vi "Write.vi"(8 "error in (no error)":errorcluster, 9 "Start address":string, 10 "Read Type":variant, 11 "MelsecTCP in":refnum<class "InovanceSerial.lvclass">) -> (0 "error out":errorcluster, 3 "MelsecTCP out":refnum<class "InovanceSerial.lvclass">)   [LabVIEW 2020, in "HslCommunication.lvlib" / "InovanceSerial.lvclass"]
uses:
  InovanceSerial.lvclass
  D:/Git/Labview-Libraries/Libraries/HslCommunication/Abstract PLC Controler/Abstract PLC Controler.lvclass
  EventLogger.lvlibp/1abvi3w/vi.lib/gpm_packages/@cs/event-logger/Source/Composed Log/Types/Log Level.ctl
  Abstract PLC Controler/Abstract PLC Controler.lvclass/Abstract PLC Controler.ctl
  D:/Git/Labview-Libraries/Libraries/HslCommunication/_Dependenciecs/HslCommunication.dll
  _Dependenciecs/HslCommunication.dll
  Read reference.vi
  Abstract PLC Controler/Abstract PLC Controler.lvclass
  InovanceSerial.lvclass/InovanceSerial.ctl
  <vilib>/Utility/Data Type/NI_Data Type.lvlib
  EventLogger.lvlibp/Logger.lvclass
  EventLogger.lvlibp/1abvi3w/vi.lib/gpm_packages/@cs/event-logger/Source/Composed Log/Composed Log.lvlib
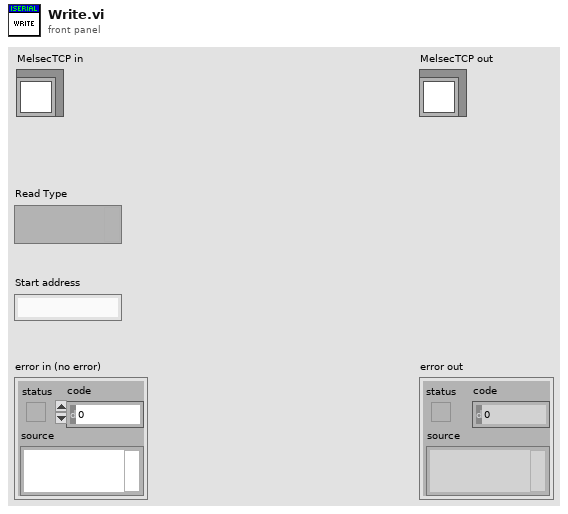
[diagram p1: front panel]
types:
  T1 = typedef "EventLogger.lvlibp/Composed Log.lvlib/Log Level.ctl" = enum16{"Debug", "Info", "Warning", "Error", "Critical"}
  T2 = typedef "NI_Data Type.lvlib/Data Type.ctl" = enum8{"Invalid Type", "Void", "I8", "I16", "I32", "I64", "U8", "U16", "U32", "U64", "Single Float", "Double Float", "Extended Float", "Single Complex", "Double Complex", "Extended Complex", "Enum U8", "Enum U16", "Enum U32", "Enum U64", "Single Float With Unit", "Double Float With Unit", "Extended Float With Unit", "Single Complex with Unit", "Double Complex with Unit", "Extended Complex with Unit", "Boolean", "String", "Path", "Picture", "Tag", "Array", "Cluster", "Variant", "LV Variant", "Waveform", "Timestamp", "Digital Waveform", "Digital Data", "ExpressData", "Refnum", "External Data", "VI", "Poly VI", "LabVIEW Class Instance", "Fixed Point", "Set Collection", "Map Collection"}
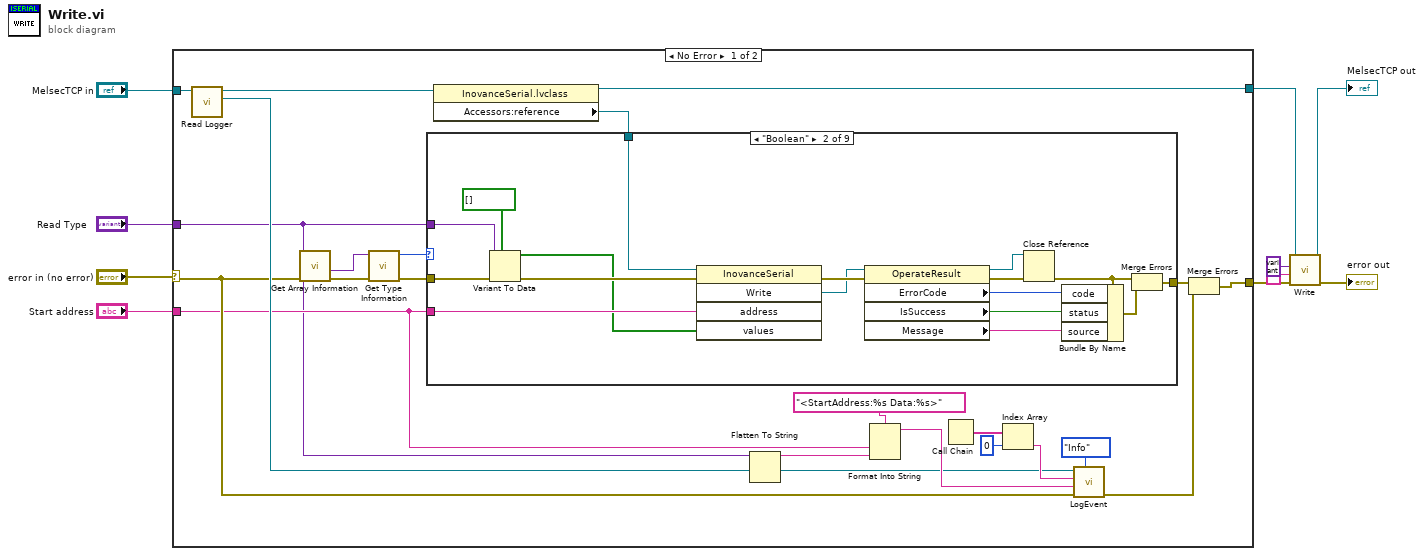
[diagram p0: block diagram]
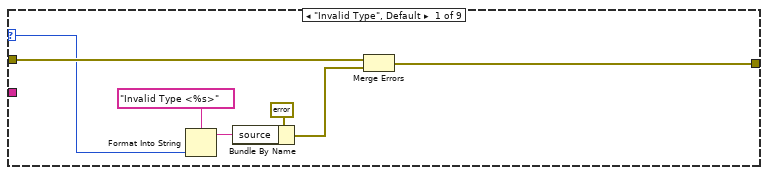
[diagram p2: hidden frame]
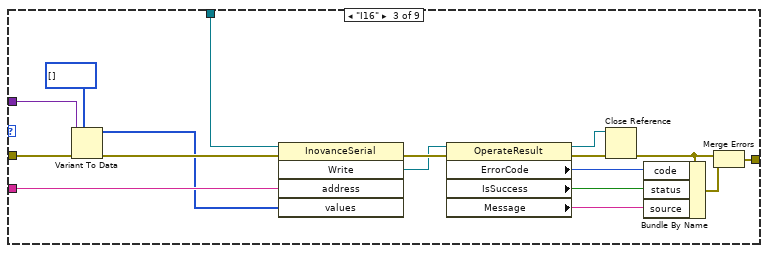
[diagram p3: hidden frame]
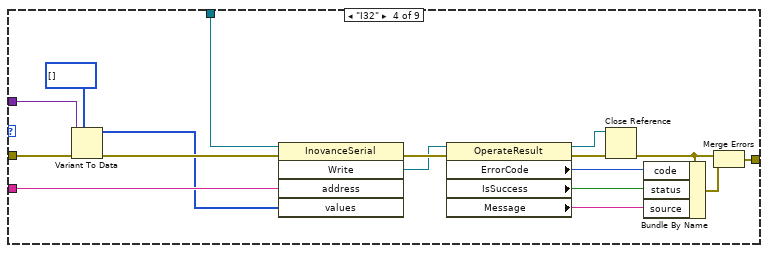
[diagram p4: hidden frame]
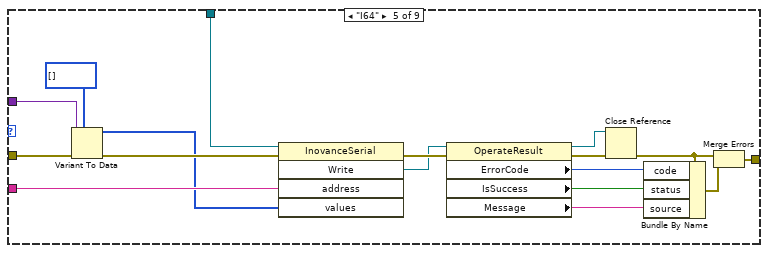
[diagram p5: hidden frame]
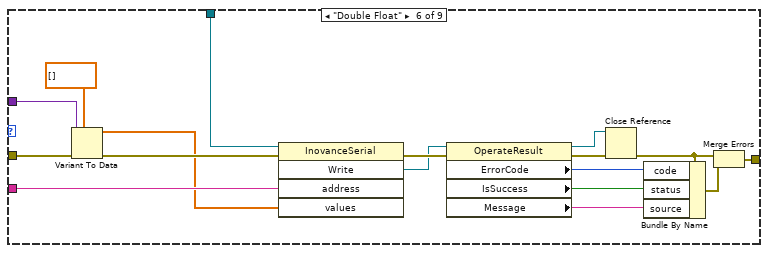
[diagram p6: hidden frame]
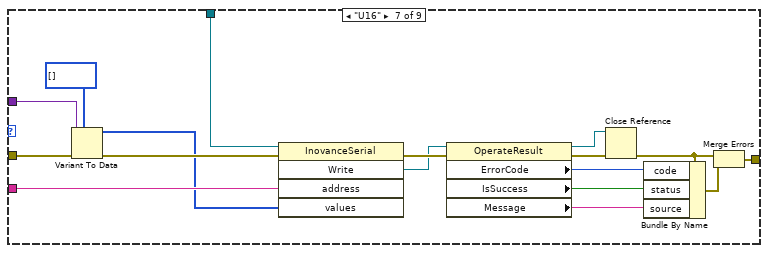
[diagram p7: hidden frame]
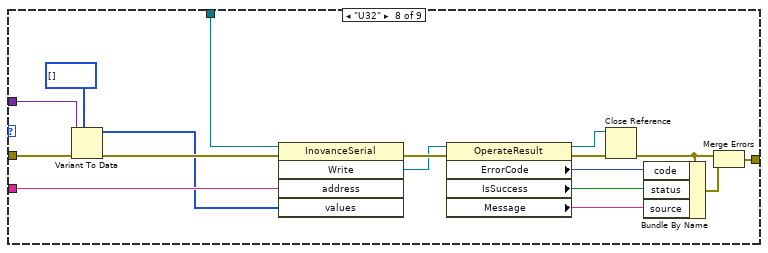
[diagram p8: hidden frame]
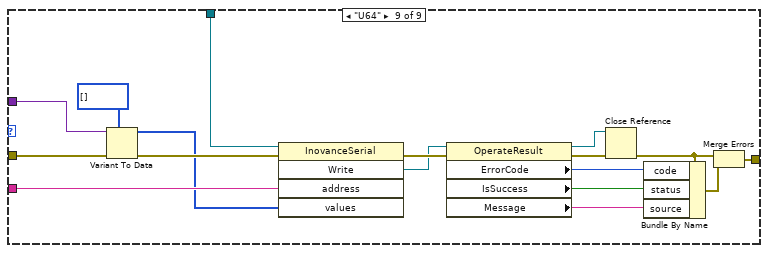
[diagram p9: hidden frame]
diagram:
  n1 = case shown="No Error" "error in (no error)" {
    selector: "error in (no error)" -> [w16 w177]
    tunnel: "MelsecTCP in" -> [w32 w176]
    tunnel: [w29 w176] -> w4
    tunnel: "Start address" -> [w15 _]
    tunnel: [w12 w177] -> w7
    tunnel: "Read Type" -> [w14 _]
    frame No Error {
      n2 = call "Read Logger.vi"("Abstract PLC Controler in"=w32) -> ("EventLogger.lvlibp:Logger.lvclass"=w17:refnum<class "Logger.lvclass">, "Abstract PLC Controler out"=w18:refnum<class "InovanceSerial.lvclass">)  [unwired: 9 in]
      n3 = call <vilib>:"Get Array Information.vi"("error in (no error)"=w16, "variant"=w14) -> ("error out"=w27:errorcluster, "array element data type"=w28:variant)  [unwired: 6 in, 2 out]
      n4 = call <vilib>:"Get Type Information.vi"("error in (no error)"=w27, "variant"=w28) -> ("error out"=w26:errorcluster, "type"=w25:T2)  [unwired: 5 in, 3 out]
      n5 = property class="InovanceSerial.lvclass"(reference=w18) -> (reference out=w29:refnum<class "InovanceSerial.lvclass">, "Accessors:reference"=w31:refnum<k24>)  [unwired: 1 in, 1 out]
      n6 = case shown="\"Boolean\"" w25 {
        selector: w25 -> [w37 _ _ _ _ _ _ _ _]
        tunnel: w31 -> [_ w56 w73 w90 w107 w124 w141 w158 w175]
        tunnel: w15 -> [_ w55 w72 w89 w106 w123 w140 w157 w174]
        tunnel: [w38 w54 w71 w88 w105 w122 w139 w156 w173] -> w30
        tunnel: w14 -> [_ w48 w65 w82 w99 w116 w133 w150 w167]
        tunnel: w26 -> [w39 w47 w64 w81 w98 w115 w132 w149 w166]
        frame "Invalid Type", Default {
          n7 = Format Into String(format string="Invalid Type <%s>", w37) -> (resulting string=w34:string)  [unwired: 2 in, 1 out]
          n8 = Bundle By Name(cluster=errorcluster {"status"=TRUE, "code"=-1, "source"=""} ("error IO"), "source"=w34) -> (w33:errorcluster)
          n9 = Merge Errors(w39, w33) -> (w38:errorcluster)
        }
        frame "Boolean" {
          n10 = Variant To Data(error in=w47, type=bool[] [], Variant=w48) -> (data=w40:bool[], error out=w42:errorcluster)
          n11 = invoke class="InovanceSerial" method="Write"(reference=w56, error in=w42, "address"=w55, "values"=w40) -> (error out=w46:errorcluster, "Write"=w44:refnum<k24>)  [unwired: 1 in, 3 out]
          n12 = property class="OperateResult"(reference=w44, error in=w46) -> (reference out=w43:refnum<k24>, error out=w45:errorcluster, "ErrorCode"=w53:i32, "IsSuccess"=w52:bool, "Message"=w51:string)
          n13 = Close Reference(reference=w43, error in (no error)=w45) -> (error out=w50:errorcluster)
          n14 = Bundle By Name(cluster=w50, "code"=w53, "status"=w52, "source"=w51) -> (w49:errorcluster)
          n15 = Merge Errors(w50, w49) -> (w54:errorcluster)
        }
        frame "I16" {
          n16 = Variant To Data(error in=w64, type=i16[] [], Variant=w65) -> (data=w57:i16[], error out=w59:errorcluster)
          n17 = invoke class="InovanceSerial" method="Write"(reference=w73, error in=w59, "address"=w72, "values"=w57) -> (error out=w63:errorcluster, "Write"=w61:refnum<k24>)  [unwired: 1 in, 3 out]
          n18 = property class="OperateResult"(reference=w61, error in=w63) -> (reference out=w60:refnum<k24>, error out=w62:errorcluster, "ErrorCode"=w70:i32, "IsSuccess"=w69:bool, "Message"=w68:string)
          n19 = Close Reference(reference=w60, error in (no error)=w62) -> (error out=w67:errorcluster)
          n20 = Bundle By Name(cluster=w67, "code"=w70, "status"=w69, "source"=w68) -> (w66:errorcluster)
          n21 = Merge Errors(w67, w66) -> (w71:errorcluster)
        }
        frame "I32" {
          n22 = Variant To Data(error in=w81, type=i32[] [], Variant=w82) -> (data=w74:i32[], error out=w76:errorcluster)
          n23 = invoke class="InovanceSerial" method="Write"(reference=w90, error in=w76, "address"=w89, "values"=w74) -> (error out=w80:errorcluster, "Write"=w78:refnum<k24>)  [unwired: 1 in, 3 out]
          n24 = property class="OperateResult"(reference=w78, error in=w80) -> (reference out=w77:refnum<k24>, error out=w79:errorcluster, "ErrorCode"=w87:i32, "IsSuccess"=w86:bool, "Message"=w85:string)
          n25 = Close Reference(reference=w77, error in (no error)=w79) -> (error out=w84:errorcluster)
          n26 = Bundle By Name(cluster=w84, "code"=w87, "status"=w86, "source"=w85) -> (w83:errorcluster)
          n27 = Merge Errors(w84, w83) -> (w88:errorcluster)
        }
        frame "I64" {
          n28 = Variant To Data(error in=w98, type=i64[] [], Variant=w99) -> (data=w91:i64[], error out=w93:errorcluster)
          n29 = invoke class="InovanceSerial" method="Write"(reference=w107, error in=w93, "address"=w106, "values"=w91) -> (error out=w97:errorcluster, "Write"=w95:refnum<k24>)  [unwired: 1 in, 3 out]
          n30 = property class="OperateResult"(reference=w95, error in=w97) -> (reference out=w94:refnum<k24>, error out=w96:errorcluster, "ErrorCode"=w104:i32, "IsSuccess"=w103:bool, "Message"=w102:string)
          n31 = Close Reference(reference=w94, error in (no error)=w96) -> (error out=w101:errorcluster)
          n32 = Bundle By Name(cluster=w101, "code"=w104, "status"=w103, "source"=w102) -> (w100:errorcluster)
          n33 = Merge Errors(w101, w100) -> (w105:errorcluster)
        }
        frame "Double Float" {
          n34 = Variant To Data(error in=w115, type=dbl[] [], Variant=w116) -> (data=w108:dbl[], error out=w110:errorcluster)
          n35 = invoke class="InovanceSerial" method="Write"(reference=w124, error in=w110, "address"=w123, "values"=w108) -> (error out=w114:errorcluster, "Write"=w112:refnum<k24>)  [unwired: 1 in, 3 out]
          n36 = property class="OperateResult"(reference=w112, error in=w114) -> (reference out=w111:refnum<k24>, error out=w113:errorcluster, "ErrorCode"=w121:i32, "IsSuccess"=w120:bool, "Message"=w119:string)
          n37 = Close Reference(reference=w111, error in (no error)=w113) -> (error out=w118:errorcluster)
          n38 = Bundle By Name(cluster=w118, "code"=w121, "status"=w120, "source"=w119) -> (w117:errorcluster)
          n39 = Merge Errors(w118, w117) -> (w122:errorcluster)
        }
        frame "U16" {
          n40 = Variant To Data(error in=w132, type=u16[] [], Variant=w133) -> (data=w125:u16[], error out=w127:errorcluster)
          n41 = invoke class="InovanceSerial" method="Write"(reference=w141, error in=w127, "address"=w140, "values"=w125) -> (error out=w131:errorcluster, "Write"=w129:refnum<k24>)  [unwired: 1 in, 3 out]
          n42 = property class="OperateResult"(reference=w129, error in=w131) -> (reference out=w128:refnum<k24>, error out=w130:errorcluster, "ErrorCode"=w138:i32, "IsSuccess"=w137:bool, "Message"=w136:string)
          n43 = Close Reference(reference=w128, error in (no error)=w130) -> (error out=w135:errorcluster)
          n44 = Bundle By Name(cluster=w135, "code"=w138, "status"=w137, "source"=w136) -> (w134:errorcluster)
          n45 = Merge Errors(w135, w134) -> (w139:errorcluster)
        }
        frame "U32" {
          n46 = Variant To Data(error in=w149, type=u32[] [], Variant=w150) -> (data=w142:u32[], error out=w144:errorcluster)
          n47 = invoke class="InovanceSerial" method="Write"(reference=w158, error in=w144, "address"=w157, "values"=w142) -> (error out=w148:errorcluster, "Write"=w146:refnum<k24>)  [unwired: 1 in, 3 out]
          n48 = property class="OperateResult"(reference=w146, error in=w148) -> (reference out=w145:refnum<k24>, error out=w147:errorcluster, "ErrorCode"=w155:i32, "IsSuccess"=w154:bool, "Message"=w153:string)
          n49 = Close Reference(reference=w145, error in (no error)=w147) -> (error out=w152:errorcluster)
          n50 = Bundle By Name(cluster=w152, "code"=w155, "status"=w154, "source"=w153) -> (w151:errorcluster)
          n51 = Merge Errors(w152, w151) -> (w156:errorcluster)
        }
        frame "U64" {
          n52 = Variant To Data(error in=w166, type=u64[] [], Variant=w167) -> (data=w159:u64[], error out=w161:errorcluster)
          n53 = invoke class="InovanceSerial" method="Write"(reference=w175, error in=w161, "address"=w174, "values"=w159) -> (error out=w165:errorcluster, "Write"=w163:refnum<k24>)  [unwired: 1 in, 3 out]
          n54 = property class="OperateResult"(reference=w163, error in=w165) -> (reference out=w162:refnum<k24>, error out=w164:errorcluster, "ErrorCode"=w172:i32, "IsSuccess"=w171:bool, "Message"=w170:string)
          n55 = Close Reference(reference=w162, error in (no error)=w164) -> (error out=w169:errorcluster)
          n56 = Bundle By Name(cluster=w169, "code"=w172, "status"=w171, "source"=w170) -> (w168:errorcluster)
          n57 = Merge Errors(w169, w168) -> (w173:errorcluster)
        }
      }
      n58 = Flatten To String(anything=w14) -> (data string=w13:string)  [unwired: 3 in, 2 out]
      n59 = Format Into String(format string="<StartAddress:%s Data:%s>", w15, w13) -> (resulting string=w21:string)  [unwired: 2 in, 1 out]
      n60 = Call Chain() -> (call chain=w24:string[])
      n61 = Index Array(array=w24, index=0) -> (element=w20:string)
      n62 = call "LogEvent.vi"("Event Level"=Log_Level."Info", "error in (no error)"=w16, "Data To Log"=w21, "SourceID"=w20, "Logger in"=w17) -> ("error out"=w11:errorcluster)  [unwired: 5 in, 1 out]
      n63 = Merge Errors(w30, w11) -> (w12:errorcluster)
    }
    frame Error {
    }
  }
  n64 = call-parent "Write.vi"("error in (no error)"=w7, "Start address"="", "Read Type"=variant, "MelsecTCP in"=w4) -> ("error out"=→"error out":errorcluster, "MelsecTCP out"=→"MelsecTCP out":refnum<class "InovanceSerial.lvclass">)  [unwired: 6 in]
